vi "Decrypt.vi"(8 "error in (no error)":errorcluster, 10 "Ciphertext":string, 11 "AES in":refnum<class "AES.lvclass">) -> (0 "error out":errorcluster, 2 "Plaintext":string, 3 "AES out":refnum<class "AES.lvclass">)   [LabVIEW 2020, in "AES.lvclass"]
uses:
  AES.lvclass
  AES.lvclass/AES.ctl
  Ton Plomp Encryption/Encryption.lvlib
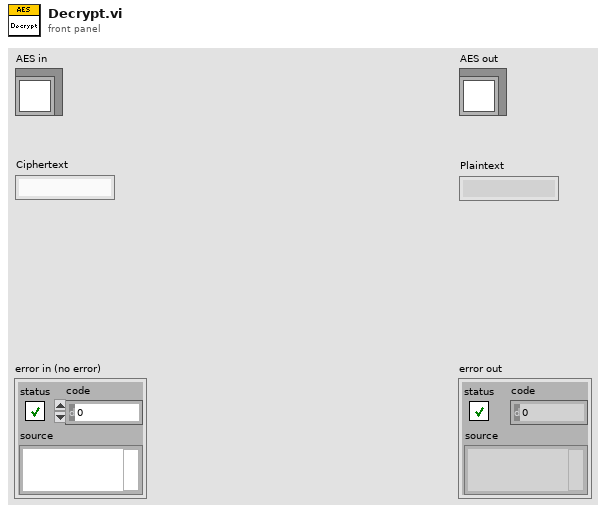
[diagram p1: front panel]
types:
  T1 = typedef "Encryption.lvlib/AES-Modes.ctl" = enum16{"ECB", "CBC", "CFB128", "OFB"}
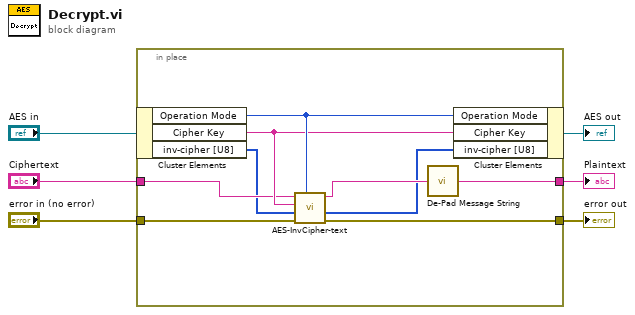
[diagram p0: block diagram]
diagram:
  n1 = in-place {
    in-place-border: "Ciphertext" -> [w13]
    in-place-border: [w12] -> w4
    in-place-border: "error in (no error)" -> [w11]
    in-place-border: [w10] -> w2
    n2 = in-place-cluster #1("AES in") -> ("Operation Mode"=w15:T1, "Cipher Key"=w14:string, "inv-cipher [U8]"=w8:u8[])
    n3 = call "AES-InvCipher-text.vi"("Operation Mode"=w15, "error in (no error)"=w11, "inv-cipher [U8]"=w8, "Cipher Key"=w14, "ciphertext"=w13) -> ("error out"=w10:errorcluster, "inv-cipher out"=w7:u8[], "plaintext"=w9:string)  [unwired: 4 in]
    n4 = call "De-Pad Message String.vi"("Padded Message In"=w9) -> ("Message Out"=w12:string)
    n5 = in-place-cluster #1("Operation Mode"=w15, "Cipher Key"=w14, "inv-cipher [U8]"=w7) -> (→"AES out":refnum<class "AES.lvclass">)
  }
  "error out" <- w2
  "Plaintext" <- w4
